vi "readTDMS.vi"(8 "error in (no error)":errorcluster, 11 "Path Out":path) -> (0 "error out":errorcluster, 3 "Array":dbl[][](array[numeric]))   [LabVIEW 2013, in "main.lvlib"]
uses:
  main.lvlib
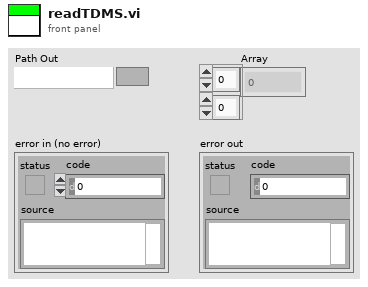
[diagram p1: front panel]
types:
  T1 = enum16{"open", "open or create", "create or replace", "create", "open (read-only)"}
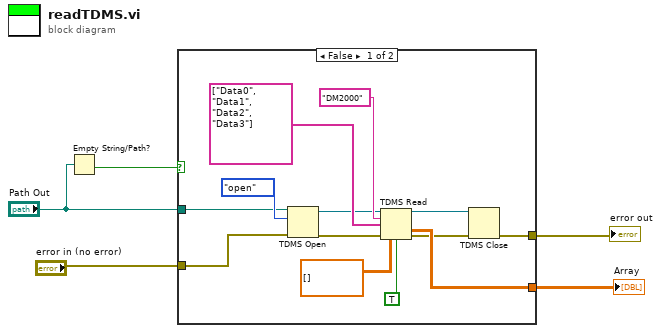
[diagram p0: block diagram]
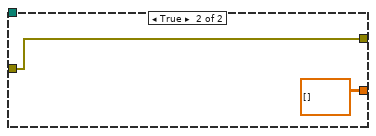
[diagram p2: hidden frame]
diagram:
  n1 = Empty String/Path?(string/path="Path Out") -> (empty?=w2:bool)
  n2 = case shown="False" w2 {
    tunnel: "error in (no error)" -> [w18 w20]
    tunnel: [w15 w20] -> w4
    tunnel: [w13 dbl[][] []] -> w3
    tunnel: "Path Out" -> [w6 _]
    frame False {
      n3 = TDMS Open(8:w18, 10:T1."open" ("operation (0:open)"), 11:w6) -> (0:w17:errorcluster, 3:w10:refnum<k34>)  [unwired: 4 in]
      n4 = TDMS Read(0:w10, 5:"DM2000" ("group name in"), 7:string[] ["Data0", "Data1", "Data2", "Data3"], 11:w17, 12:dbl[][] [], 13:TRUE ("return channels in file order? (F)")) -> (4:w8:refnum<k34>, 10:w13:dbl[][], 15:w9:errorcluster)  [unwired: 2 in, 3 out]
      n5 = TDMS Close(8:w9, 11:w8) -> (0:w15:errorcluster)  [unwired: 1 out]
    }
    frame True {
    }
  }
  "error out" <- w4
  "Array" <- w3
